vi "aes_decryptor.vi"(1 "Encrypted":string, 2 "Key":string) -> (0 "Decrypted":string)   [LabVIEW 2017]
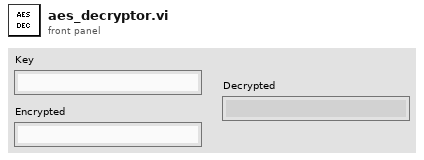
[diagram p1: front panel]
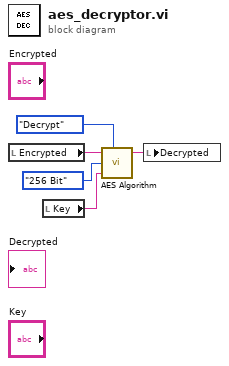
[diagram p0: block diagram]
diagram:
  n1 = local read "Encrypted"() -> (w4:string)
  n2 = local read "Key"() -> (w5:string)
  n3 = call "AES Algorithm.vi"("Input"=w4, "Mode"=enum16{"Encrypt", "Decrypt"}."Decrypt", "KeySize"=enum16{"128 Bit", "192 Bit", "256 Bit"}."256 Bit", "Key (128 Bit)"=w5) -> ("Output"=w3:string)  [unwired: 4 in, 1 out]
  n4 = local write "Decrypted"(w3) -> ()
